vi "Abstract_Function_to_Boolean_Hierarchy.vi"   [LabVIEW 2021]
uses:
  One Term/SGL/AbsComp_One Term_SGL.lvclass
  One Term/CPLX_SGL/AbsComp_One Term_CPLX_SGL.lvclass
  One Term/DBL/AbsComp_One Term_DBL.lvclass
  One Term/EXT/AbsComp_One Term_EXT.lvclass
  One Term/CPLX_DBL/AbsComp_One Term_CPLX_DBL.lvclass
  One Term/CPLX_EXT/AbsComp_One Term_CPLX_EXT.lvclass
  One Term/I8/AbsComp_One Term_I8.lvclass
  One Term/I16/AbsComp_One Term_I16.lvclass
  One Term/I32/AbsComp_One Term_I32.lvclass
  One Term/I64/AbsComp_One Term_I64.lvclass
  One Term/U8/AbsComp_One Term_U8.lvclass
  One Term/U16/AbsComp_One Term_U16.lvclass
  One Term/U32/AbsComp_One Term_U32.lvclass
  One Term/U64/AbsComp_One Term_U64.lvclass
  One Term/Time/AbsComp_One Term_Time.lvclass
  One Term/STR/AbsComp_One Term_STR.lvclass
  Two Term/Bool/AbsComp_Two Term_Bool.lvclass
  Two Term/STR/AbsComp_Two Term_STR.lvclass
  Two Term/SGL/AbsComp_Two Term_SGL.lvclass
  Two Term/DBL/AbsComp_Two Term_DBL.lvclass
  Two Term/EXT/AbsComp_Two Term_EXT.lvclass
  Two Term/CPLX_DBL/AbsComp_Two Term_CPLX_DBL.lvclass
  Two Term/CPLX_SGL/AbsComp_Two Term_CPLX_SGL.lvclass
  Two Term/CPLX_EXT/AbsComp_Two Term_CPLX_EXT.lvclass
  Two Term/I8/AbsComp_Two Term_I8.lvclass
  Two Term/I16/AbsComp_Two Term_I16.lvclass
  Two Term/I32/AbsComp_Two Term_I32.lvclass
  Two Term/I64/AbsComp_Two Term_I64.lvclass
  Two Term/U8/AbsComp_Two Term_U8.lvclass
  Two Term/U16/AbsComp_Two Term_U16.lvclass
  Two Term/U32/AbsComp_Two Term_U32.lvclass
  Two Term/U64/AbsComp_Two Term_U64.lvclass
  Two Term/Time/AbsComp_Two Term_Time.lvclass
  Abs_Types/Boolean/Abs_Boolean.lvclass
panel:
  # "SEE DIAGRAM\nFOR Hierarchy"
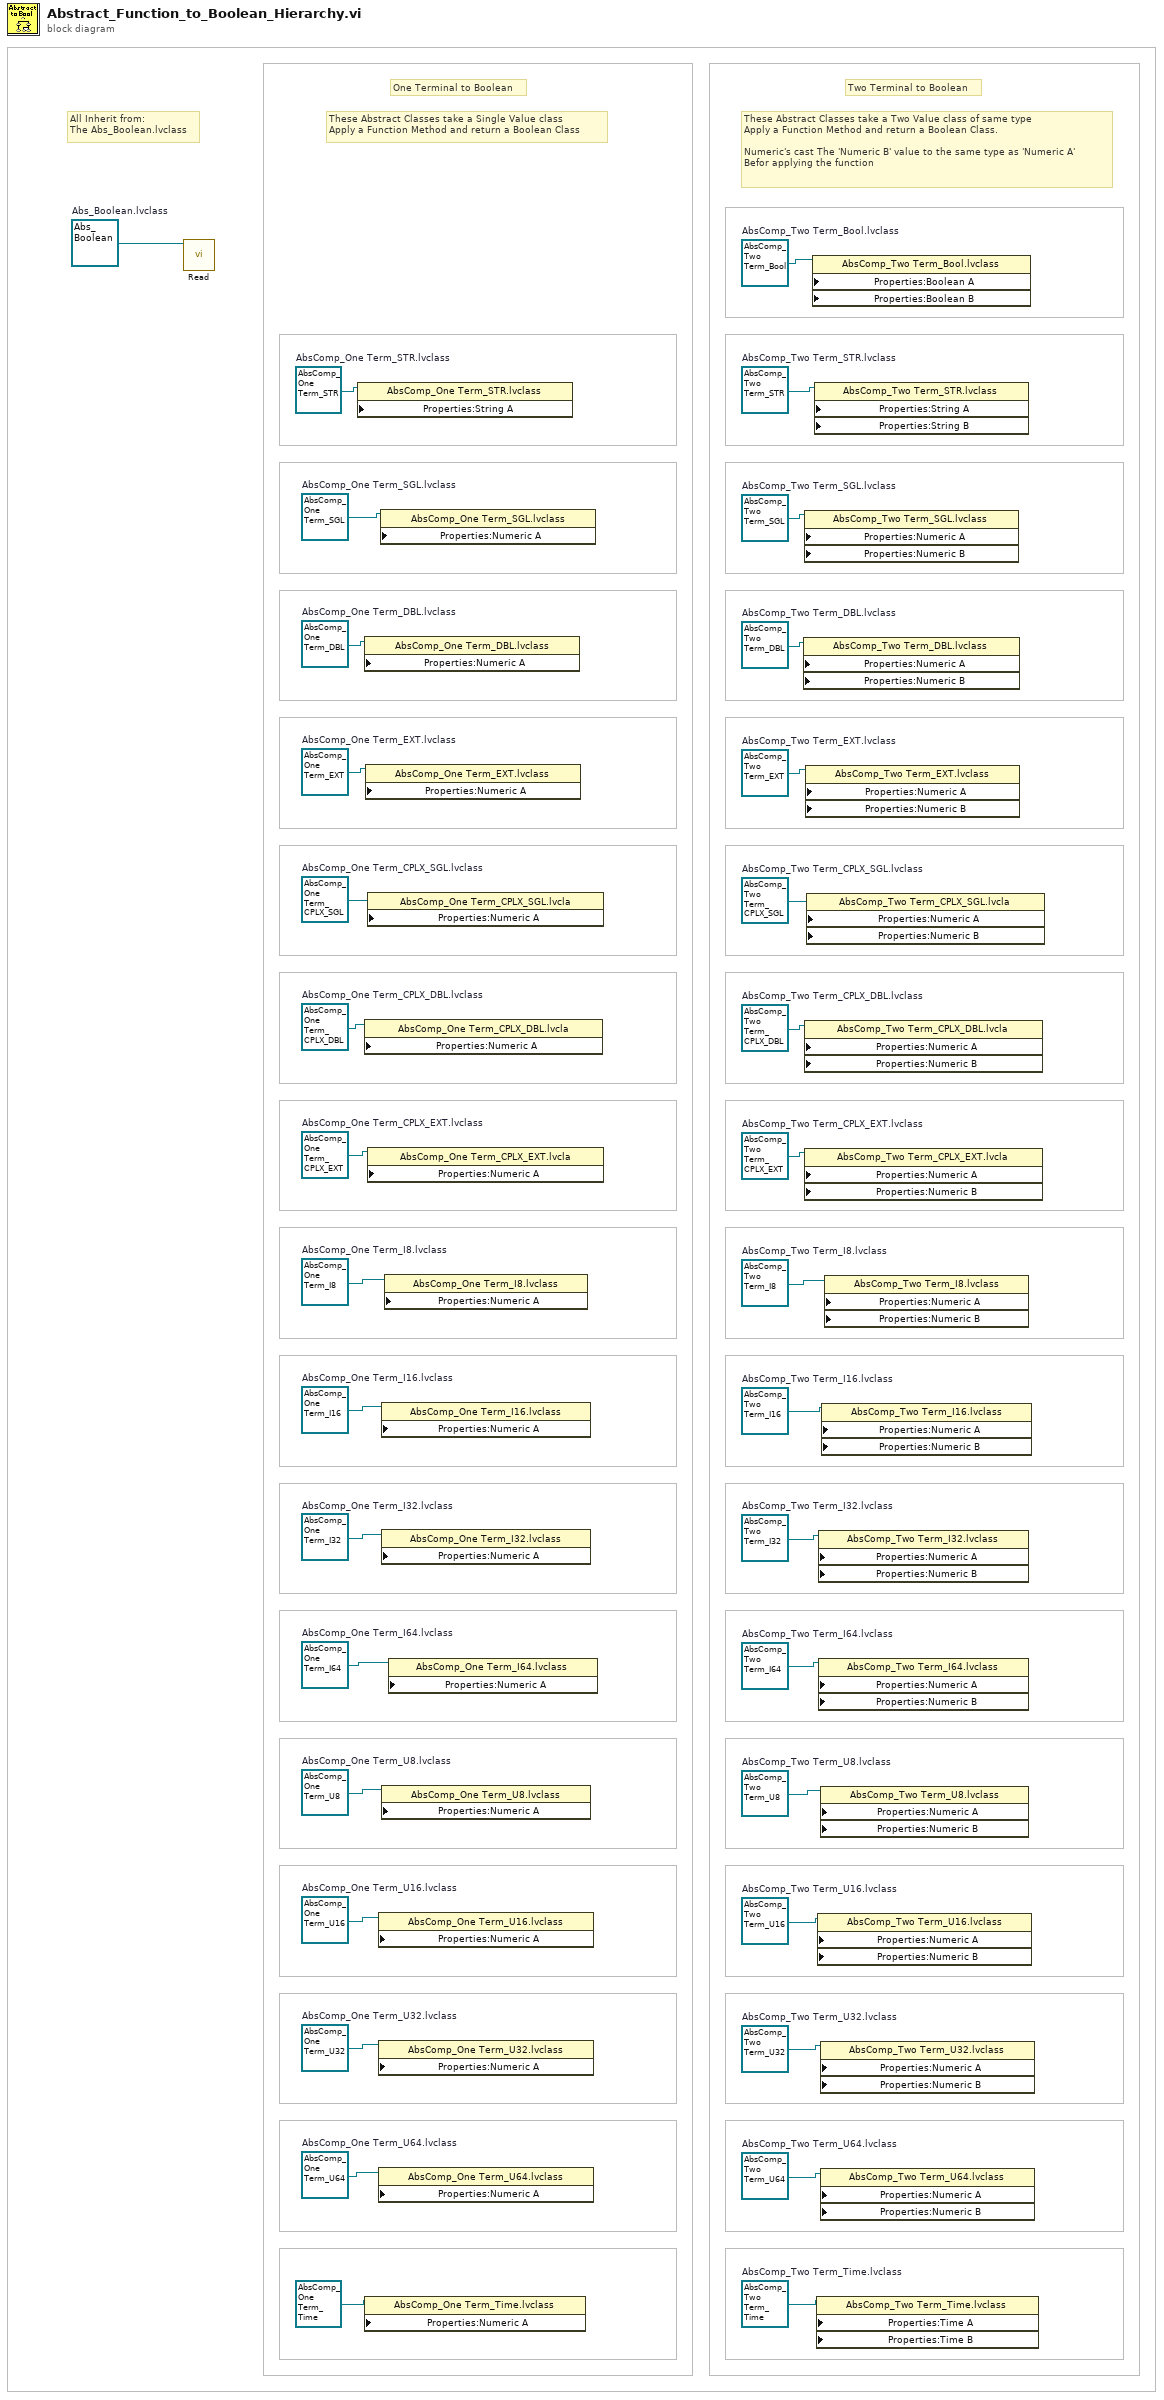
[diagram p0: block diagram]
diagram:
  w1 = refnum<class "Abs_Boolean.lvclass"> refnum  # Abs_Boolean.lvclass
  w2 = refnum<class "AbsComp_Two Term_Time.lvclass"> refnum  # AbsComp_Two Term_Time.lvclass
  w3 = refnum<class "AbsComp_Two Term_U64.lvclass"> refnum  # AbsComp_Two Term_U64.lvclass
  w4 = refnum<class "AbsComp_Two Term_U32.lvclass"> refnum  # AbsComp_Two Term_U32.lvclass
  w5 = refnum<class "AbsComp_Two Term_U16.lvclass"> refnum  # AbsComp_Two Term_U16.lvclass
  w6 = refnum<class "AbsComp_Two Term_U8.lvclass"> refnum  # AbsComp_Two Term_U8.lvclass
  w7 = refnum<class "AbsComp_Two Term_I64.lvclass"> refnum  # AbsComp_Two Term_I64.lvclass
  w8 = refnum<class "AbsComp_Two Term_I32.lvclass"> refnum  # AbsComp_Two Term_I32.lvclass
  w9 = refnum<class "AbsComp_Two Term_I16.lvclass"> refnum  # AbsComp_Two Term_I16.lvclass
  w10 = refnum<class "AbsComp_Two Term_I8.lvclass"> refnum  # AbsComp_Two Term_I8.lvclass
  w11 = refnum<class "AbsComp_Two Term_CPLX_EXT.lvclass"> refnum  # AbsComp_Two Term_CPLX_EXT.lvclass
  w13 = refnum<class "AbsComp_Two Term_CPLX_SGL.lvclass"> refnum  # AbsComp_Two Term_CPLX_SGL.lvclass
  w12 = refnum<class "AbsComp_Two Term_CPLX_DBL.lvclass"> refnum  # AbsComp_Two Term_CPLX_DBL.lvclass
  w14 = refnum<class "AbsComp_Two Term_EXT.lvclass"> refnum  # AbsComp_Two Term_EXT.lvclass
  w15 = refnum<class "AbsComp_Two Term_DBL.lvclass"> refnum  # AbsComp_Two Term_DBL.lvclass
  w16 = refnum<class "AbsComp_Two Term_SGL.lvclass"> refnum  # AbsComp_Two Term_SGL.lvclass
  w17 = refnum<class "AbsComp_Two Term_STR.lvclass"> refnum  # AbsComp_Two Term_STR.lvclass
  w18 = refnum<class "AbsComp_Two Term_Bool.lvclass"> refnum  # AbsComp_Two Term_Bool.lvclass
  w19 = refnum<class "AbsComp_One Term_STR.lvclass"> refnum  # AbsComp_One Term_STR.lvclass
  w29 = refnum<class "AbsComp_One Term_U64.lvclass"> refnum  # AbsComp_One Term_U64.lvclass
  w28 = refnum<class "AbsComp_One Term_U32.lvclass"> refnum  # AbsComp_One Term_U32.lvclass
  w27 = refnum<class "AbsComp_One Term_U16.lvclass"> refnum  # AbsComp_One Term_U16.lvclass
  w26 = refnum<class "AbsComp_One Term_U8.lvclass"> refnum  # AbsComp_One Term_U8.lvclass
  w25 = refnum<class "AbsComp_One Term_I64.lvclass"> refnum  # AbsComp_One Term_I64.lvclass
  w24 = refnum<class "AbsComp_One Term_I32.lvclass"> refnum  # AbsComp_One Term_I32.lvclass
  w23 = refnum<class "AbsComp_One Term_I16.lvclass"> refnum  # AbsComp_One Term_I16.lvclass
  w22 = refnum<class "AbsComp_One Term_I8.lvclass"> refnum  # AbsComp_One Term_I8.lvclass
  w21 = refnum<class "AbsComp_One Term_CPLX_EXT.lvclass"> refnum  # AbsComp_One Term_CPLX_EXT.lvclass
  w30 = refnum<class "AbsComp_One Term_CPLX_DBL.lvclass"> refnum  # AbsComp_One Term_CPLX_DBL.lvclass
  w31 = refnum<class "AbsComp_One Term_EXT.lvclass"> refnum  # AbsComp_One Term_EXT.lvclass
  w32 = refnum<class "AbsComp_One Term_DBL.lvclass"> refnum  # AbsComp_One Term_DBL.lvclass
  w33 = refnum<class "AbsComp_One Term_CPLX_SGL.lvclass"> refnum  # AbsComp_One Term_CPLX_SGL.lvclass
  w34 = refnum<class "AbsComp_One Term_SGL.lvclass"> refnum  # AbsComp_One Term_SGL.lvclass
  # "All Inherit from: \nThe Abs_Boolean.lvclass"
  # "These Abstract Classes take a Two Value class of same type\nApply a Function Method and return a Boolean Class.\n\nNumeric's cast The 'Numeric B' value to the same type as 'Numeric A'\nBefor applying the function"
  # "These Abstract Classes take a Single Value class\nApply a Function Method and return a Boolean Class"
  # "One Terminal to Boolean"
  # "Two Terminal to Boolean"
  n1 = call-dynamic "Read.vi"("Boolean in"=w1) -> ()  [unwired: 8 in, 3 out]
  n2 = property class="AbsComp_One Term_STR.lvclass" props=["Properties:String A"](reference=w19) -> ()  [unwired: 2 in, 2 out]
  n3 = property class="AbsComp_One Term_DBL.lvclass" props=["Properties:Numeric A"](reference=w32) -> ()  [unwired: 2 in, 2 out]
  n4 = property class="AbsComp_One Term_CPLX_DBL.lvcla" props=["Properties:Numeric A"](reference=w30) -> ()  [unwired: 2 in, 2 out]
  n5 = property class="AbsComp_One Term_Time.lvclass" props=["Properties:Numeric A"](reference=refnum<class "AbsComp_One Term_Time.lvclass"> refnum ("AbsComp_One Term_Time.lvclass")) -> ()  [unwired: 2 in, 2 out]
  n6 = property class="AbsComp_One Term_EXT.lvclass" props=["Properties:Numeric A"](reference=w31) -> ()  [unwired: 2 in, 2 out]
  n7 = property class="AbsComp_One Term_CPLX_SGL.lvcla" props=["Properties:Numeric A"](reference=w33) -> ()  [unwired: 2 in, 2 out]
  n8 = property class="AbsComp_One Term_CPLX_EXT.lvcla" props=["Properties:Numeric A"](reference=w21) -> ()  [unwired: 2 in, 2 out]
  n9 = property class="AbsComp_One Term_U16.lvclass" props=["Properties:Numeric A"](reference=w27) -> ()  [unwired: 2 in, 2 out]
  n10 = property class="AbsComp_One Term_U32.lvclass" props=["Properties:Numeric A"](reference=w28) -> ()  [unwired: 2 in, 2 out]
  n11 = property class="AbsComp_One Term_U64.lvclass" props=["Properties:Numeric A"](reference=w29) -> ()  [unwired: 2 in, 2 out]
  n12 = property class="AbsComp_One Term_SGL.lvclass" props=["Properties:Numeric A"](reference=w34) -> ()  [unwired: 2 in, 2 out]
  n13 = property class="AbsComp_One Term_I16.lvclass" props=["Properties:Numeric A"](reference=w23) -> ()  [unwired: 2 in, 2 out]
  n14 = property class="AbsComp_One Term_I32.lvclass" props=["Properties:Numeric A"](reference=w24) -> ()  [unwired: 2 in, 2 out]
  n15 = property class="AbsComp_One Term_U8.lvclass" props=["Properties:Numeric A"](reference=w26) -> ()  [unwired: 2 in, 2 out]
  n16 = property class="AbsComp_One Term_I8.lvclass" props=["Properties:Numeric A"](reference=w22) -> ()  [unwired: 2 in, 2 out]
  n17 = property class="AbsComp_One Term_I64.lvclass" props=["Properties:Numeric A"](reference=w25) -> ()  [unwired: 2 in, 2 out]
  n18 = property class="AbsComp_Two Term_DBL.lvclass" props=["Properties:Numeric A", "Properties:Numeric B"](reference=w15) -> ()  [unwired: 3 in, 2 out]
  n19 = property class="AbsComp_Two Term_SGL.lvclass" props=["Properties:Numeric A", "Properties:Numeric B"](reference=w16) -> ()  [unwired: 3 in, 2 out]
  n20 = property class="AbsComp_Two Term_CPLX_DBL.lvcla" props=["Properties:Numeric A", "Properties:Numeric B"](reference=w12) -> ()  [unwired: 3 in, 2 out]
  n21 = property class="AbsComp_Two Term_CPLX_EXT.lvcla" props=["Properties:Numeric A", "Properties:Numeric B"](reference=w11) -> ()  [unwired: 3 in, 2 out]
  n22 = property class="AbsComp_Two Term_EXT.lvclass" props=["Properties:Numeric A", "Properties:Numeric B"](reference=w14) -> ()  [unwired: 3 in, 2 out]
  n23 = property class="AbsComp_Two Term_CPLX_SGL.lvcla" props=["Properties:Numeric A", "Properties:Numeric B"](reference=w13) -> ()  [unwired: 3 in, 2 out]
  n24 = property class="AbsComp_Two Term_Bool.lvclass" props=["Properties:Boolean A", "Properties:Boolean B"](reference=w18) -> ()  [unwired: 3 in, 2 out]
  n25 = property class="AbsComp_Two Term_STR.lvclass" props=["Properties:String A", "Properties:String B"](reference=w17) -> ()  [unwired: 3 in, 2 out]
  n26 = property class="AbsComp_Two Term_Time.lvclass" props=["Properties:Time A", "Properties:Time B"](reference=w2) -> ()  [unwired: 3 in, 2 out]
  n27 = property class="AbsComp_Two Term_U16.lvclass" props=["Properties:Numeric A", "Properties:Numeric B"](reference=w5) -> ()  [unwired: 3 in, 2 out]
  n28 = property class="AbsComp_Two Term_I32.lvclass" props=["Properties:Numeric A", "Properties:Numeric B"](reference=w8) -> ()  [unwired: 3 in, 2 out]
  n29 = property class="AbsComp_Two Term_I64.lvclass" props=["Properties:Numeric A", "Properties:Numeric B"](reference=w7) -> ()  [unwired: 3 in, 2 out]
  n30 = property class="AbsComp_Two Term_U8.lvclass" props=["Properties:Numeric A", "Properties:Numeric B"](reference=w6) -> ()  [unwired: 3 in, 2 out]
  n31 = property class="AbsComp_Two Term_U32.lvclass" props=["Properties:Numeric A", "Properties:Numeric B"](reference=w4) -> ()  [unwired: 3 in, 2 out]
  n32 = property class="AbsComp_Two Term_U64.lvclass" props=["Properties:Numeric A", "Properties:Numeric B"](reference=w3) -> ()  [unwired: 3 in, 2 out]
  n33 = property class="AbsComp_Two Term_I16.lvclass" props=["Properties:Numeric A", "Properties:Numeric B"](reference=w9) -> ()  [unwired: 3 in, 2 out]
  n34 = property class="AbsComp_Two Term_I8.lvclass" props=["Properties:Numeric A", "Properties:Numeric B"](reference=w10) -> ()  [unwired: 3 in, 2 out]
